vi "postep.vi"(2 "kolejne powtórzenie pętli":i32, 3 "Całość do przetworzenia":i32) -> (0 "Proces przetwarzania zdjęć":dbl, 1 "Postęp":string)   [LabVIEW 2009]
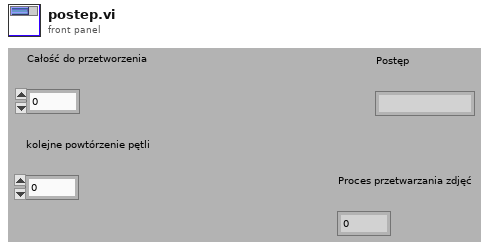
[diagram p1: front panel]
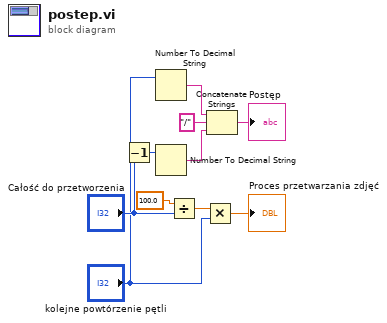
[diagram p0: block diagram]
diagram:
  n1 = Decrement(x="Całość do przetworzenia") -> (x-1=w1:i32)
  n2 = Number To Decimal String(number="kolejne powtórzenie pętli") -> (decimal integer string=w7:string)  [unwired: 1 in]
  n3 = Number To Decimal String(number=w1) -> (decimal integer string=w6:string)  [unwired: 1 in]
  n4 = Divide(x=100.0, y="Całość do przetworzenia") -> (x/y=w3:dbl)
  n5 = Multiply(x=w3, y="kolejne powtórzenie pętli") -> (x*y=→"Proces przetwarzania zdjęć":dbl)
  n6 = Concatenate Strings(w7, "/" ("string"), w6) -> (→"Postęp":string)
